vi "0~1随机数发生器1D（dbl).vi"(8 "Error In":errorcluster caption="错误输入", 10 "Length":i32) -> (0 "Error Out":errorcluster caption="错误输出", 3 "Rand(0~1) 1D":dbl[](array[numeric]))   [LabVIEW 2013]
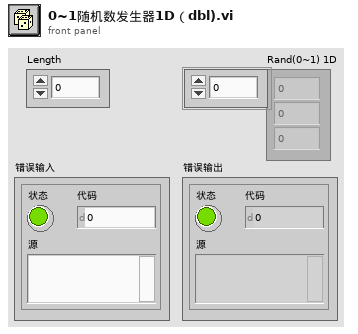
[diagram p1: front panel]
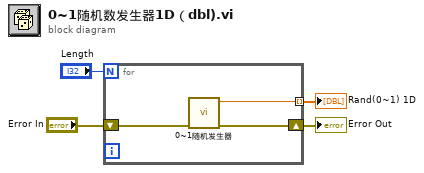
[diagram p0: block diagram]
diagram:
  n1 = for {
    N: "Length" -> [_]
    shift-right: [w6] -> w3
    shift-left: "Error In" -> [w7]
    tunnel: [w5] -> w2 mode=indexing
    n2 = call-poly "0~1随机发生器.vi"("Error In"=w7) -> ("Error Out"=w6:errorcluster, "Rand(0-1)"=w5:dbl)  [unwired: 9 in]
  }
  "Error Out" <- w3
  "Rand(0~1) 1D" <- w2
